vi "setUp.vi"(8 "error in (no error)":errorcluster, 11 "reference in":refnum<class "Test mysql.lvclass">=refnum) -> (0 "error out":errorcluster, 3 "reference out":refnum<class "Test mysql.lvclass">)   [LabVIEW 2020, in "DataBase_mysql_Tests.lvlib" / "Test mysql.lvclass"]
doc: "setUp runs prior to the test method during test execution. Use this method to initialize any object data required by your tests."
uses:
  Test mysql.lvclass
  C:/Program Files/National Instruments/LabVIEW 2020/vi.lib/addons/_JKI Toolkits/VI Tester/TestCase.llb/TestCase.lvclass
  externals/mysql/Source/mysql.net/mysql.lvclass
  Test mysql.lvclass/Test mysql.ctl
  695df06e-9ac4-443d-876f-6906eb82b222.vi
  <vilib>/Utility/error.llb/Error Cluster From Error Code.vi
  <vilib>/addons/_JKI Toolkits/VI Tester/TestCase.llb/TestCase.lvclass
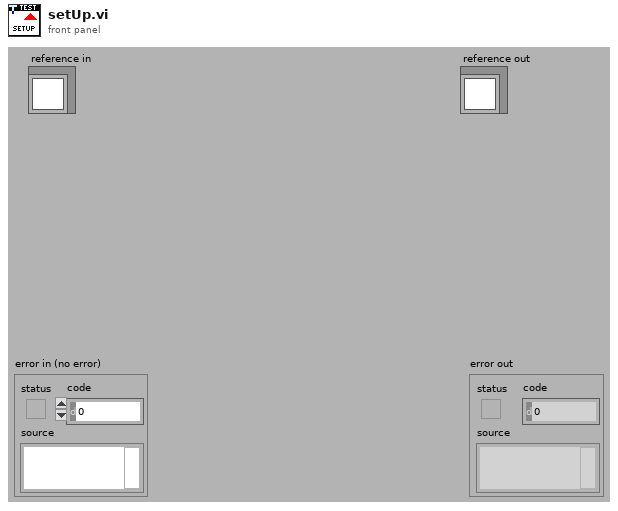
[diagram p1: front panel]
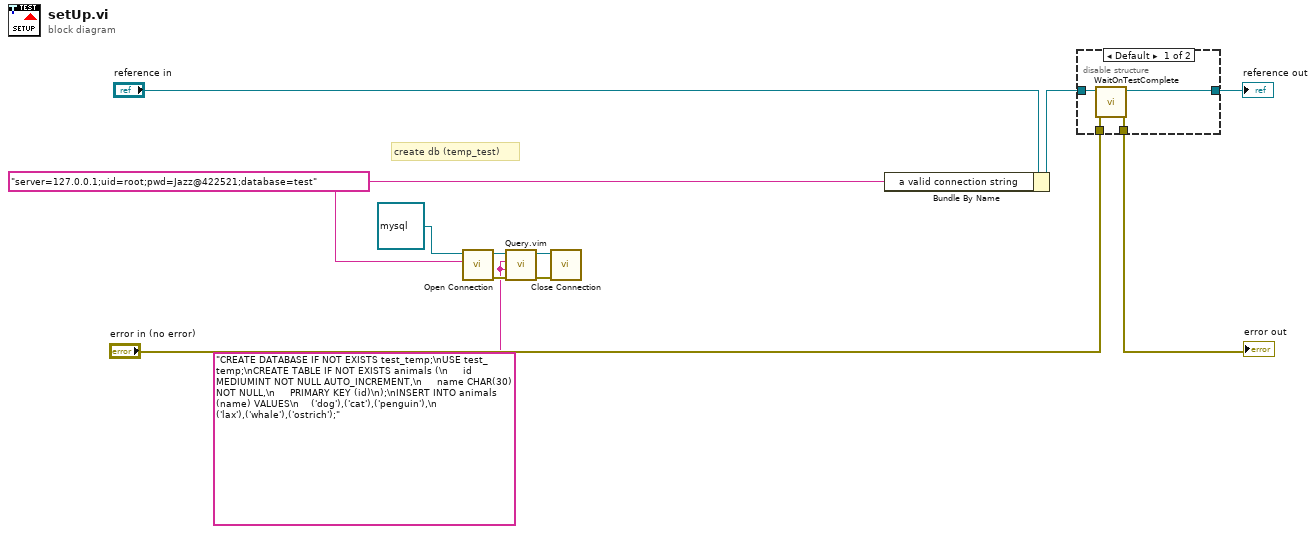
[diagram p0: block diagram]
diagram:
  w6 = "server=127.0.0.1;uid=root;pwd=Jazz@422521;database=test" ("a valid connection string")
  w1 = "CREATE DATABASE IF NOT EXISTS test_temp;\nUSE test_temp;\nCREATE TABLE IF NOT EXISTS animals (\n     id MEDIUMINT NOT NULL AUTO_INCREMENT,\n     name CHAR(30) NOT NULL,\n     PRIMARY KEY (id)\n);\nINSERT INTO animals (name) VALUES\n    ('dog'),('cat'),('penguin'),\n    ('lax'),('whale'),('ostrich');"
  # "create db (temp_test)"
  n1 = call-dynamic "Open Connection.vi"("Connection string"=w6, "mysql in"=refnum<class "mysql.lvclass"> refnum) -> ("error out"=w3:errorcluster, "mysql out"=w5:refnum<class "mysql.lvclass">)  [unwired: 8 in]
  n2 = call "Query.vim"("error in (no error)"=w3, "Type and Default"=w1, "Query string"=w1, "IDatabase in"=w5) -> ("error out"=w2:errorcluster, "IDatabase out"=w4:refnum<class "mysql.lvclass">)  [unwired: 5 in, 1 out]
  n3 = call-dynamic "Close Connection.vi"("error in (no error)"=w2, "mysql in"=w4) -> ()  [unwired: 8 in, 2 out]
  n4 = Bundle By Name(cluster="reference in", "a valid connection string"=w6) -> (w8:refnum<class "Test mysql.lvclass">)
  n5 = disable-structure shown="Default" {
    disable-tunnel: "error in (no error)" -> [w16 w17]
    disable-tunnel: [w15 w17] -> w11
    disable-tunnel: [w14 w18] -> w9
    disable-tunnel: w8 -> [w13 w18]
    frame condition #0 (active) {
      n6 = call <vilib>:"WaitOnTestComplete.vi"("error in (no error)"=w16, "TestCase in"=w13) -> ("error out"=w15:errorcluster, "TestCase out"=w14:refnum<class "Test mysql.lvclass">)  [unwired: 8 in]
    }
    frame condition #1 {
    }
  }
  "error out" <- w11
  "reference out" <- w9
